vi "Open SMO.vi"(8 "error in (no error)":errorcluster, 11 "Instrument in":refnum<class "Instrument.lvclass">) -> (0 "error out":errorcluster, 3 "Instrument out":refnum<class "Instrument.lvclass">)   [LabVIEW 2019, in "Instrument.lvlib" / "Instrument.lvclass"]
uses:
  Instrument.lvclass
  Instrument.lvclass/Instrument.ctl
  <userlib>/LevyLab/RemoteControl/RemoteControl/RemoteControl.lvclass
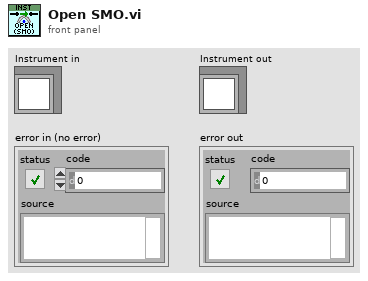
[diagram p1: front panel]
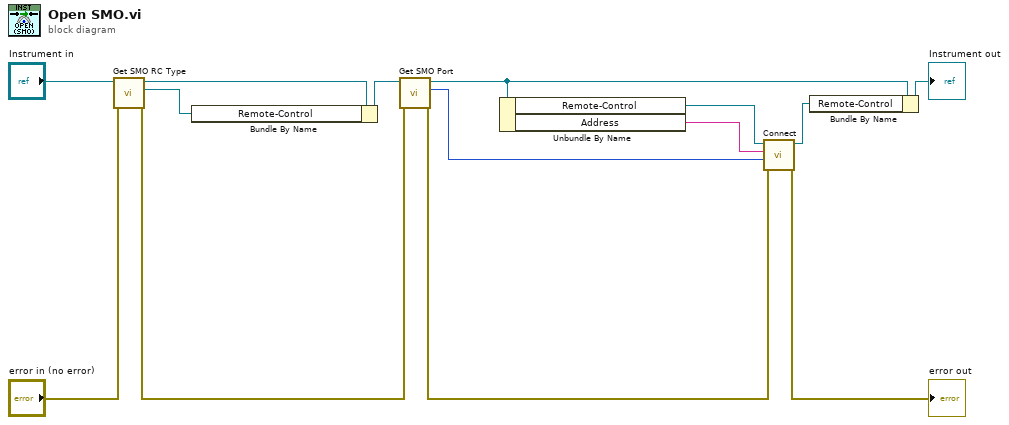
[diagram p0: block diagram]
diagram:
  n1 = call-dynamic "Get SMO RC Type.vi"("error in (no error)"="error in (no error)", "Instrument in"="Instrument in") -> ("error out"=w6:errorcluster, "RemoteControl"=w3:refnum<class "RemoteControl.lvclass">, "Instrument out"=w2:refnum<class "Instrument.lvclass">)  [unwired: 7 in]
  n2 = Bundle By Name(cluster=w2, "Remote-Control"=w3) -> (w1:refnum<class "Instrument.lvclass">)
  n3 = call-dynamic "Get SMO Port.vi"("error in (no error)"=w6, "Instrument in"=w1) -> ("error out"=w14:errorcluster, "Port"=w5:u16, "Instrument out"=w13:refnum<class "Instrument.lvclass">)  [unwired: 7 in]
  n4 = Unbundle By Name(w13) -> ("Remote-Control"=w9:refnum<class "RemoteControl.lvclass">, "Address"=w4:string)
  n5 = call <userlib>:"Connect.vi"("error in (no error)"=w14, "Port"=w5, "address"=w4, "RemoteControl in"=w9) -> ("error out"=→"error out":errorcluster, "RemoteControl out"=w10:refnum<class "RemoteControl.lvclass">)  [unwired: 6 in]
  n6 = Bundle By Name(cluster=w13, "Remote-Control"=w10) -> (→"Instrument out":refnum<class "Instrument.lvclass">)
